vi "p1.vi"() -> ()   [LabVIEW 2023, in "d22.lvlib"]
uses:
  d22.lvlib
  AOC/AOC.lvlib
panel:
  out "size(s)":i32=375
  in  "Example":string="1,0,1~1,2,1\n0,0,2~2,0,2\n0,2,3~2,2,3\n0,0,4~0,2,4\n2,0,5~2,2,5\n0,1,6~2,1,6\n1,1,8~1,1,9"
  in  "Example":bool
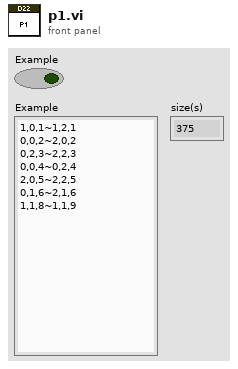
[diagram p1: front panel]
types:
  T1 = cluster{"max":cluster{"x":i32, "y":i32, "z":i32}, "min":cluster{"x":i32, "y":i32, "z":i32}, "supported by":i32[], "supporting":i32[]}
  T2 = cluster{"max":cluster{"x":i32, "y":i32, "z":i32}, "min":cluster{"x":i32, "y":i32, "z":i32}, "supported by":i32[], "supporting":i32[]}[]
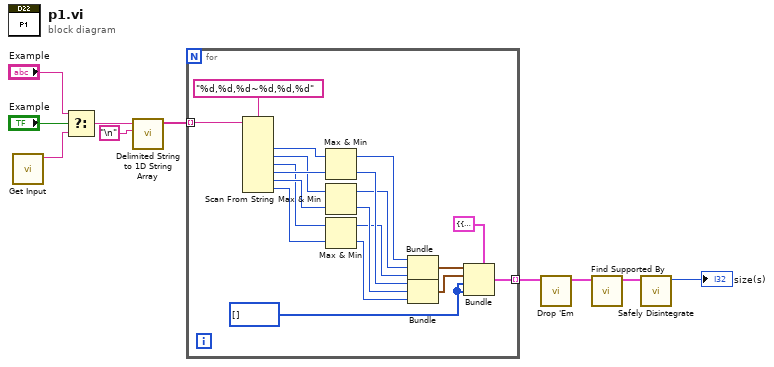
[diagram p0: block diagram]
diagram:
  n1 = call "Get Input.vi"() -> ("Input"=w10:string)  [unwired: 11 in]
  n2 = Select(t="Example", s="Example", f=w10) -> (s? t:f=w9:string)
  n3 = call <vilib>:"Delimited String to 1D String Array.vi"("delimiter"="\n", "delimited string"=w9) -> ("string array"=w6:string[])  [unwired: 9 in]
  n4 = for {
    tunnel: w6 -> [w29] mode=indexing
    tunnel: [w27] -> w5 mode=indexing
    w11 = i32[] [] ("supports")
    n5 = Scan From String(format string="%d,%d,%d~%d,%d,%d", input string=w29) -> (output 1=w25:i32, output 2=w23:i32, output 3=w21:i32, output 4=w24:i32, output 5=w22:i32, output 6=w20:i32)  [unwired: 8 in, 3 out]
    n6 = Max & Min(x=w25, y=w24) -> (max(x,y)=w15:i32, min(x,y)=w16:i32)
    n7 = Max & Min(x=w23, y=w22) -> (max(x,y)=w14:i32, min(x,y)=w17:i32)
    n8 = Max & Min(x=w21, y=w20) -> (max(x,y)=w13:i32, min(x,y)=w18:i32)
    n9 = Bundle(w15, w14, w13) -> (w28:cluster{i32, i32, i32})  [unwired: 1 in]
    n10 = Bundle(w16, w17, w18) -> (w19:cluster{i32, i32, i32})  [unwired: 1 in]
    n11 = Bundle(cluster=T1 {"max"={"x"=0, "y"=0, "z"=0}, "min"={"x"=0, "y"=0, "z"=0}, "supported by"=[], "supporting"=[]}, "max"=w28, "min"=w19, "supported by"=w11, "supporting"=w11) -> (w27:T1)
  }
  n12 = call "Drop 'Em.vi"("Bricks in"=w5) -> ("Bricks out"=w3:T2)  [unwired: 10 in]
  n13 = call "Find Supported By.vi"("Bricks in"=w3) -> ("Bricks out"=w2:T2)  [unwired: 10 in]
  n14 = call "Safely Disintegrate.vi"("Bricks in"=w2) -> ("Number Disintegrated"=→"size(s)":i32)  [unwired: 10 in]
